vi "8-Hide&Show MainFrontPanel.vi"(8 "error in (no error)":errorcluster, 10 "Hide&Show":enum16{"Hide", "Show"}(ring), 11 "This VI":refnum<vi>) -> (0 "error out":errorcluster)   [LabVIEW 2017]
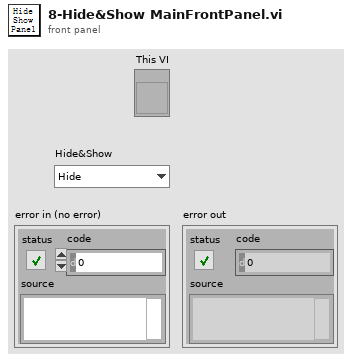
[diagram p1: front panel]
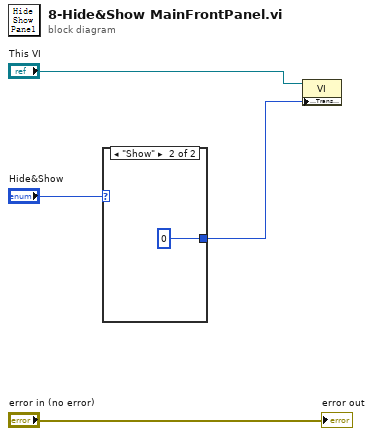
[diagram p0: block diagram]
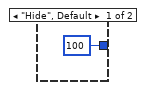
[diagram p2: hidden frame]
diagram:
  n1 = case shown="\"Show\"" "Hide&Show" {
    tunnel: [100 0] -> w1
    frame "Hide", Default {
    }
    frame "Show" {
    }
  }
  n2 = property class="VI"(reference="This VI", "FP:Transparency"=w1) -> ()  [unwired: 1 in, 2 out]
  "error out" <- "error in (no error)"
